vi "Change All Descriptions.vi"(6 "Prompt?":bool, 9 "New":string, 10 "Path":path, 11 "VI Data":T1[](array[typedef])) -> (1 "Changed Indices":i32[](array[numeric]), 2 "Adjusted All?":bool, 3 "VI Data out":T1[](array[typedef]))   [LabVIEW 2023, in "VI Properties Editor.lvlib"]
doc: "Changes the descriptions of all VIs whose name matches the one located at <B>Path</B>, to the value <B>New</B>."
uses:
  VI Properties Editor.lvlib
  CTLs/VI Data.ctl
  CTLs/VI Properties.ctl
  <vilib>/picture/picture.llb/imagedata.ctl
  CTLs/Control Properties.ctl
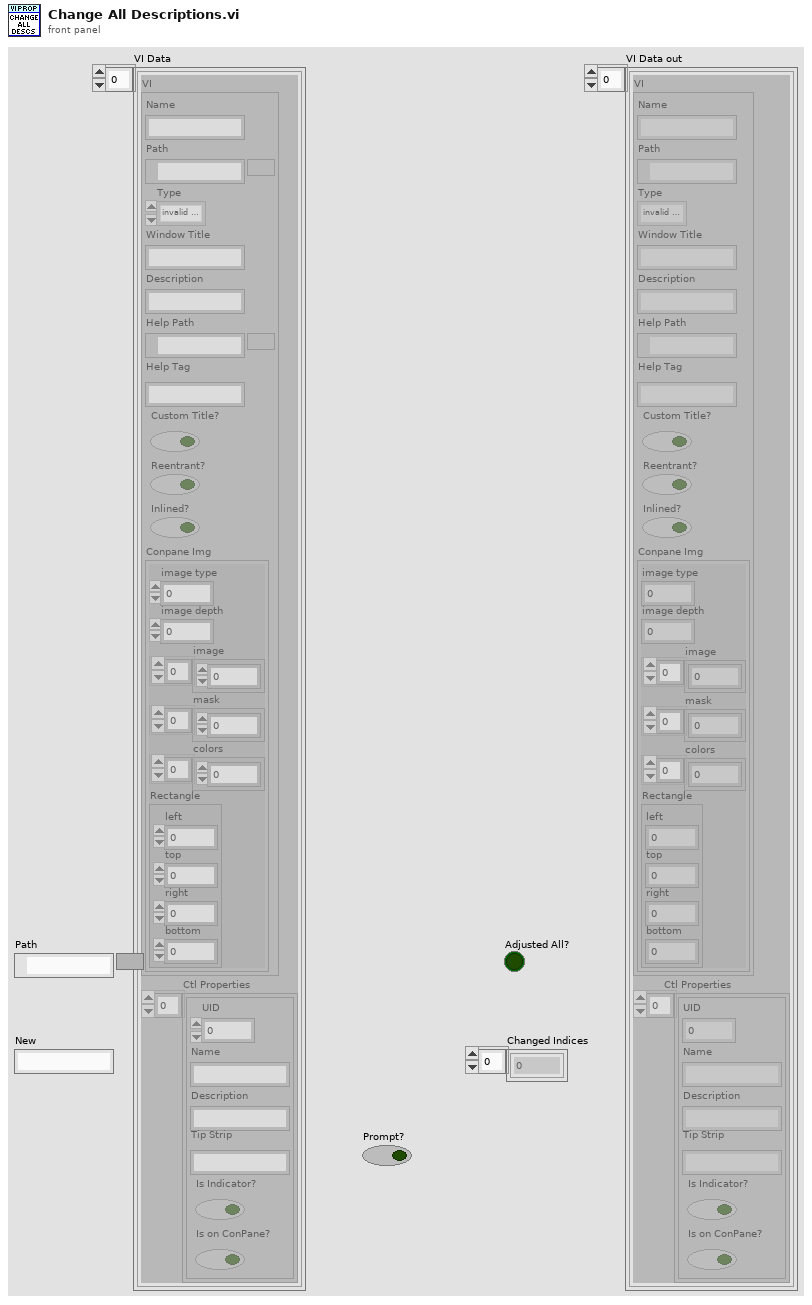
[diagram p1: front panel]
types:
  T1 = typedef "VI Properties Editor.lvlib/VI Data.ctl" = cluster{"VI":T2, "Ctl Properties":T4[]}
  T2 = typedef "VI Properties Editor.lvlib/VI Properties.ctl" = cluster{"Name":string, "Path":path, "Type":enum32{"invalid VI type", "Standard VI", "Control VI", "Global VI", "Polymorphic VI", "Configuration VI", "SubSystem", "Facade VI", "Method VI", "Statechart Diagram VI"}, "Window Title":string, "Description":string, "Help Path":path, "Help Tag":string, "Custom Title?":bool, "Reentrant?":bool, "Inlined?":bool, "Conpane Img":T3}
  T3 = typedef "imagedata.ctl" = cluster{"image type":i32, "image depth":i32, "image":u8[], "mask":u8[], "colors":u32[], "Rectangle":cluster{"left":i16, "top":i16, "right":i16, "bottom":i16}}
  T4 = typedef "VI Properties Editor.lvlib/Control Properties.ctl" = cluster{"UID":i32, "Name":string, "Description":string, "Tip Strip":string, "Is Indicator?":bool, "Is on ConPane?":bool}
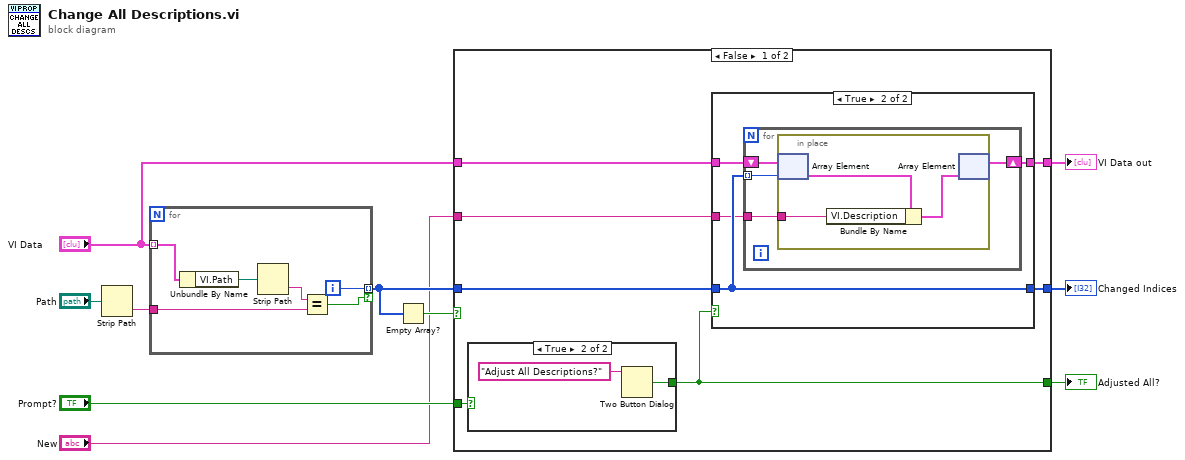
[diagram p0: block diagram]
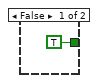
[diagram p2: hidden frame]
diagram:
  n1 = Strip Path(path="Path") -> (name=w9:string)  [unwired: 1 out]
  n2 = for {
    tunnel: "VI Data" -> [w12] mode=indexing
    tunnel: w9 -> [w16]
    tunnel: [w14] -> w5 mode=indexing if=w13
    i -> [w14]
    n3 = Unbundle By Name(w12) -> ("VI.Path"=w11:path)
    n4 = Strip Path(path=w11) -> (name=w15:string)  [unwired: 1 out]
    n5 = Equal?(x=w15, y=w16) -> (x = y?=w13:bool)
  }
  n6 = Empty Array?(array=w5) -> (empty?=w7:bool)
  n7 = case shown="False" w7 {
    tunnel: "VI Data" -> [w22 w39]
    tunnel: [w21 w39] -> w6
    tunnel: w5 -> [w23 _]
    tunnel: "Prompt?" -> [w20 _]
    tunnel: "New" -> [w17 _]
    tunnel: [w19 _] -> w2
    tunnel: [w18 _] -> w1
    frame False {
      n8 = case shown="True" w20 {
        tunnel: [TRUE ("T button?") w25] -> w18
        frame False {
        }
        frame True {
          n9 = Two Button Dialog(message="Adjust All Descriptions?") -> (T button?=w25:bool)  [unwired: 2 in]
        }
      }
      n10 = case shown="True" w18 {
        tunnel: w23 -> [_ w29]
        tunnel: w22 -> [w27 w31]
        tunnel: [w27 w30] -> w21
        tunnel: [_ w29] -> w19
        tunnel: w17 -> [_ w28]
        frame False {
        }
        frame True {
          n11 = for {
            tunnel: w29 -> [w35] mode=indexing
            shift-right: [w34] -> w30
            shift-left: w31 -> [w33]
            tunnel: w28 -> [w32]
            n12 = in-place {
              in-place-border: w32 -> [w37]
              n13 = in-place-array #1(w33, w35) -> (w38:T1)
              n14 = Bundle By Name(cluster=w38, "VI.Description"=w37) -> (w36:T1)
              n15 = in-place-array #1(w36) -> (w34:T1[])  [unwired: 1 out]
            }
          }
        }
      }
    }
    frame True {
    }
  }
  "VI Data out" <- w6
  "Changed Indices" <- w2
  "Adjusted All?" <- w1
